vi "Error message.vi"() -> ()   [LabVIEW 2020, in "NI_PID__autopid compat.lvlib"]
uses:
  <vilib>/addons/control/pid/NI_PID__autopid compat.lvlib
panel:
  in  "message":string="Only one PID loop may be tuned at a time.  You have attempted to autotune a second PID loop while the Autotuning Wizard is still in use for the first PID loop."
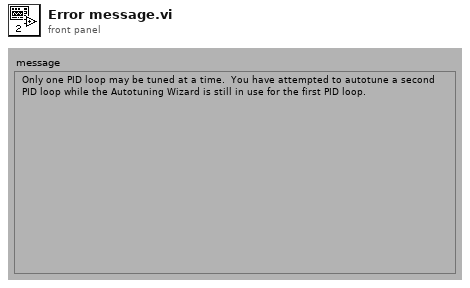
[diagram p1: front panel]
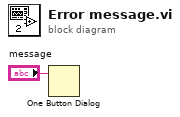
[diagram p0: block diagram]
diagram:
  n1 = One Button Dialog(message="message") -> ()  [unwired: 2 out]
